vi "Strings Levenshtein Distance.vi"(1 "String 2":string="kitten", 2 "String 1":string="sitting") -> (0 "distance":u8=3)   [LabVIEW 2010]
doc: "This VI computes the Leventshein distance between two strings.\nIt is based on the pseudocode found in Wikipedia online:\nhttp://en.wikipedia.org/wiki/Levenshtein_distance\n\n\"The Levenshtein distance between two strings is given by the minimum number of operations needed to transform one string into the other, where an operation is an insertion, deletion, or substitution of a single character.\"\n\nIt functions by creating a step matrix which is N+1 x M+1, where N and M are the lengths of the two strings to be compared, and filling in each cell of this matrix indicating how many steps (insertions, deletions, character substitutions) are required. The total number of steps to convert one string into the other is given by the last cell in the matrix.\n\nLeif S. Kirschenbaum\nMay, 2008"
uses:
  <vilib>/Analysis/1siggen.llb/Ramp Pattern by Samples.vi
  <vilib>/Analysis/NI_AALBase.lvlib
panel:
  out "step matrix":u8[][](array[numeric])=[[0, 1, 2, 3, 4, 5, 6], [1, 1, 2, 3, 4, 5, 6], [2, 2, 1, 2, 3, 4, 5], [3, 3, 2, 1, 2, 3, 4], [4, 4, 3, 2, 1, 2, 3], [5, 5, 4, 3, 2, 2, 3], [6, 6, 5, 4, 3, 3, 2], [7, 7, 6, 5, 4, 4, 3]]
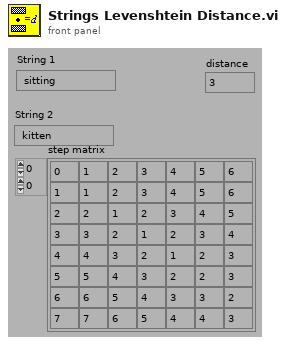
[diagram p1: front panel]
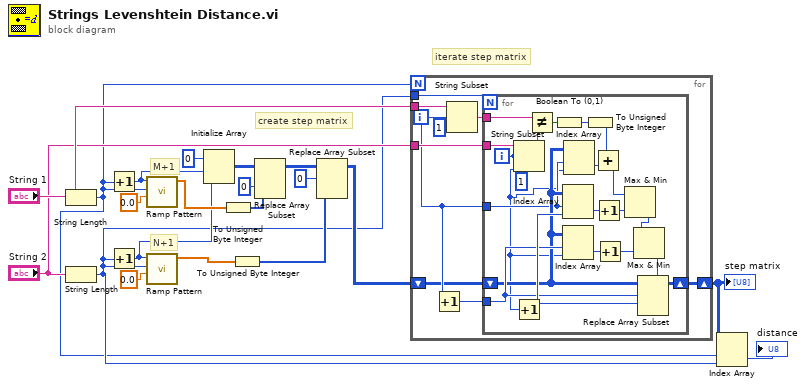
[diagram p0: block diagram]
diagram:
  # "N+1"
  # "M+1"
  # "create step matrix"
  # "iterate step matrix"
  n1 = String Length(string="String 1") -> (length=w1:i32)
  n2 = String Length(string="String 2") -> (length=w2:i32)
  n3 = Increment(x=w1) -> (x+1=w5:i32)
  n4 = Increment(x=w2) -> (x+1=w4:i32)
  n5 = call-poly <vilib>:"Ramp Pattern.vi"("start"=0.0, "end"=w1, "samples"=w5) -> ("Ramp Pattern"=w16:dbl[])  [unwired: 7 in, 1 out]
  n6 = call-poly <vilib>:"Ramp Pattern.vi"("start"=0.0, "end"=w2, "samples"=w4) -> ("Ramp Pattern"=w12:dbl[])  [unwired: 7 in, 1 out]
  n7 = Initialize Array(u8 0 ("element"), w5, w4) -> (w18:u8[][])
  n8 = To Unsigned Byte Integer(number=w16) -> (unsigned 8bit integer=w14:u8[])
  n9 = To Unsigned Byte Integer(number=w12) -> (unsigned 8bit integer=w10:u8[])
  n10 = Replace Array Subset(array=w18, new element=w14, index (col)=0 ("disabled index (col)")) -> (w13:u8[][])  [unwired: 1 in]
  n11 = Replace Array Subset(array=w13, new element=w10, index (row)=0) -> (w7:u8[][])  [unwired: 1 in]
  n12 = for {
    N: w1 -> [_]
    tunnel: "String 1" -> [w29]
    tunnel: "String 2" -> [w26]
    tunnel: w2 -> [w23]
    shift-right: [w21] -> w6
    shift-left: w7 -> [w22]
    i -> [w24]
    n13 = Increment(x=w24) -> (x+1=w25:i32)
    n14 = String Subset(string=w29, offset (0)=w24, length (rest)=1 ("length (rest)")) -> (substring=w27:string)
    n15 = for {
      N: w23 -> [_]
      tunnel: w27 -> [w47]
      tunnel: w26 -> [w49]
      tunnel: w25 -> [w41]
      tunnel: w24 -> [w32]
      shift-right: [w36] -> w21
      shift-left: w22 -> [w33]
      i -> [w31]
      n16 = String Subset(string=w49, offset (0)=w31, length (rest)=1 ("length (rest)")) -> (substring=w46:string)
      n17 = Increment(x=w31) -> (x+1=w44:i32)
      n18 = Not Equal?(x=w47, y=w46) -> (x != y?=w45:bool)
      n19 = Boolean To (0,1)(Boolean=w45) -> (0, 1=w42:i16)
      n20 = Index Array(array=w33, index (row)=w32, index (col)=w44) -> (element=w40:u8)
      n21 = Index Array(array=w33, index (row)=w41, index (col)=w31) -> (element=w39:u8)
      n22 = Index Array(array=w33, index (row)=w32, index (col)=w31) -> (element=w34:u8)
      n23 = To Unsigned Byte Integer(number=w42) -> (unsigned 8bit integer=w35:u8)
      n24 = Add(x=w35, y=w34) -> (x+y=w30:u8)
      n25 = Increment(x=w40) -> (x+1=w38:u8)
      n26 = Increment(x=w39) -> (x+1=w37:u8)
      n27 = Max & Min(x=w30, y=w38) -> (min(x,y)=w48:u8)  [unwired: 1 out]
      n28 = Max & Min(x=w48, y=w37) -> (min(x,y)=w43:u8)  [unwired: 1 out]
      n29 = Replace Array Subset(array=w33, new element=w43, index (row)=w41, index (col)=w44) -> (w36:u8[][])
    }
  }
  "step matrix" <- w6
  n30 = Index Array(array=w6, index (row)=w1, index (col)=w2) -> (element=→"distance":u8)
